vi "Bind To Type - Broken Class - Returns Error.vi"() -> ()   [LabVIEW 2017, in "Default Serialization Binder Tests.lvlib"]
uses:
  Default Serialization Binder Tests.lvlib
  Default Serialization Binder/Default Serialization Binder.lvclass
  <vilib>/addons/_JKI Toolkits/Caraya/classes/Assert/Assert Error.vi
  <vilib>/addons/_JKI Toolkits/Caraya/classes/Test/Test.lvclass
  <vilib>/addons/_JKI Toolkits/Caraya/classes/Assert/Assert.lvclass
panel:
  out "error out":errorcluster
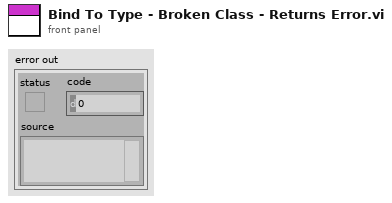
[diagram p1: front panel]
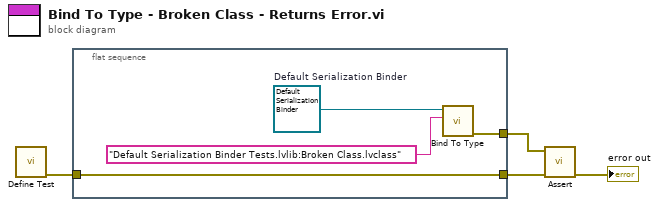
[diagram p0: block diagram]
diagram:
  n1 = call <vilib>:"Define Test.vi"() -> ("error out"=w2:errorcluster)  [unwired: 11 in]
  n2 = flat-sequence {
    tunnel: [w6] -> w3
    tunnel: w2 -> [w6]
    tunnel: [w5] -> w1
    frame #0 {
      w8 = refnum<class "Default Serialization Binder.lvclass"> refnum  # Default Serialization Binder
      n3 = call-dynamic "Bind To Type.vi"("Type Name"="Default Serialization Binder Tests.lvlib:Broken Class.lvclass", "Default Serialization Binder in"=w8) -> ("error out"=w5:errorcluster)  [unwired: 7 in, 2 out]
    }
  }
  n4 = call-poly <vilib>:"Assert.vi"("error in (no error)"=w3, "Error?"=w1) -> ("error out"=→"error out":errorcluster)  [unwired: 9 in]
